vi "Motion Profile Call VI.vi"(6 "Synchronication":enum16{"Start", "Wait"}(ring)=enum."Wait", 8 "Command Info In":T1) -> (0 "Command Info Out":T1)   [LabVIEW 2017]
uses:
  <vilib>/Rock Robotics/WPI/Framework/Command Status Info.ctl
  <vilib>/Rock Robotics/WPI/Framework/Completion Status.ctl
  <vilib>/Rock Robotics/WPI/Framework/Completion Notifier.ctl
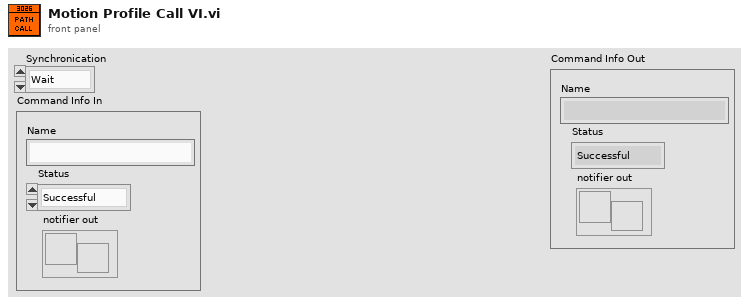
[diagram p1: front panel]
types:
  T1 = typedef "Command Status Info.ctl" = cluster{"Name":string, "Status":T2, "notifier out":T3}
  T2 = typedef "Completion Status.ctl" = enum16{"Successful", "Aborted", "Incomplete"}
  T3 = typedef "Completion Notifier.ctl" = refnum<notifier>
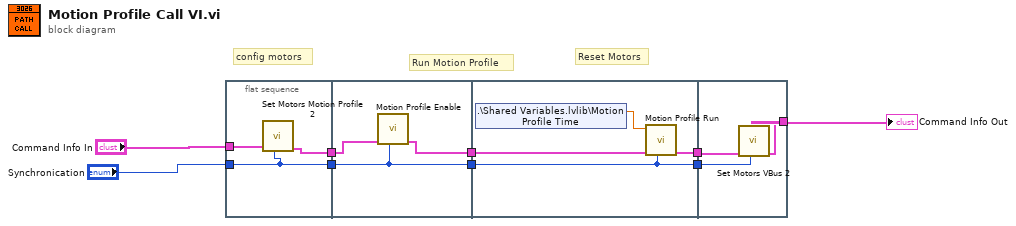
[diagram p0: block diagram]
diagram:
  # "config motors"
  # "Reset Motors"
  # "Run Motion Profile"
  n1 = flat-sequence {
    tunnel: "Command Info In" -> [w11]
    tunnel: "Synchronication" -> [w12]
    tunnel: [w12] -> w4
    tunnel: [w10] -> w2
    tunnel: w4 -> [w14]
    tunnel: [w14] -> w3
    tunnel: w2 -> [w15]
    tunnel: [w13] -> w1
    tunnel: [w19] -> w6
    tunnel: w3 -> [w17]
    tunnel: w1 -> [w18]
    tunnel: [w17] -> w5
    tunnel: [w20] -> w8
    tunnel: w6 -> [w22]
    tunnel: w5 -> [w21]
    frame #0 {
      n2 = call "Set Motors Motion Profile 2.vi"("Synchronication"=w12, "Command Info In"=w11) -> ("Command Info Out"=w10:T1)  [unwired: 9 in]
    }
    frame #1 {
      n3 = call "Motion Profile Enable.vi"("Synchronication"=w14, "Command Info In"=w15) -> ("Command Info Out"=w13:T1)  [unwired: 9 in]
    }
    frame #2 {
      n4 = shared-variable ".\\Shared Variables.lvlib\\Motion Profile Time"() -> (w16:dbl)  [unwired: 1 in, 1 out]
      n5 = call "Motion Profile Run.vi"("Synchronication"=w17, "Command Info In"=w18, "Duration"=w16) -> ("Command Info Out"=w19:T1)  [unwired: 8 in]
    }
    frame #3 {
      n6 = call "Set Motors VBus 2.vi"("Synchronication"=w21, "Command Info In"=w22) -> ("Command Info Out"=w20:T1)  [unwired: 9 in]
    }
  }
  "Command Info Out" <- w8
